vi "APC_9049_MODBUSTCP_HealingLoop.vi"() -> ()   [LabVIEW 2020]
doc: "This example demonstrates the procedure required to apply different NI-DAQmx Custom Scales to each virtual channel in a task. A DAQmx Task Property Node (Functions >> NI Measurements >> DAQmx - Data Acquisition >> DAQmx Advanced Task Options) is used to obtain the task's virtual channels. A DAQmx Channel Property Node (Functions >> NI Measurements >> DAQmx - Data Acquisition) is then used to set the custom scale for each virtual channel in the task.\n\nThe \"DAQmx Create Scale\" VI creates a custom scale for each channel in the channel list. *Note, make sure your Minimum and Maximum channel parameters are consistent with the range the scale will create."
uses:
  <vilib>/Modbus/master/Create Master Instance (TCP).vi
  <vilib>/Modbus/master/Modbus Master.lvclass
panel:
  in  "Slave address":string="172.22.11.1"
  out "register values":u16[](array[numeric])
  out "coil values":bool[](array[boolean])
  in  "Modbus STOP":bool
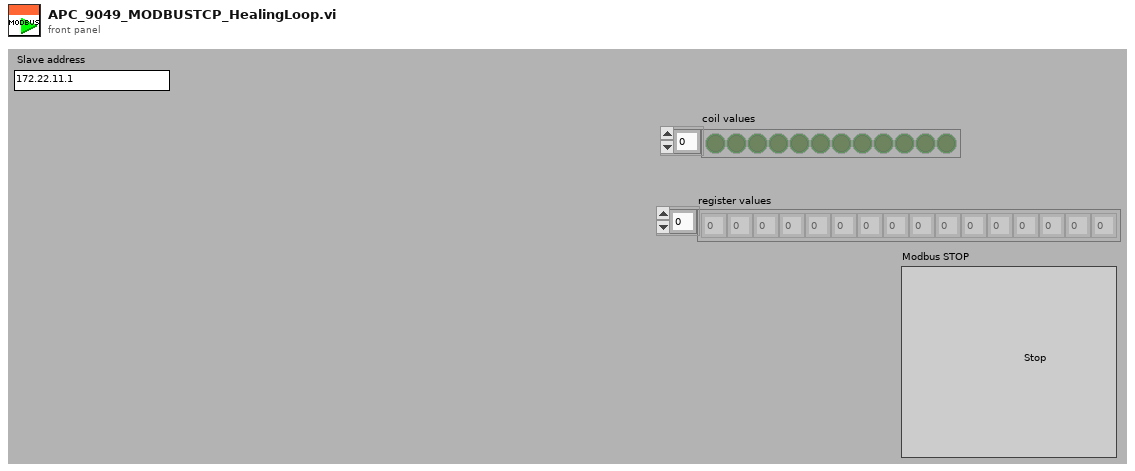
[diagram p1: front panel]
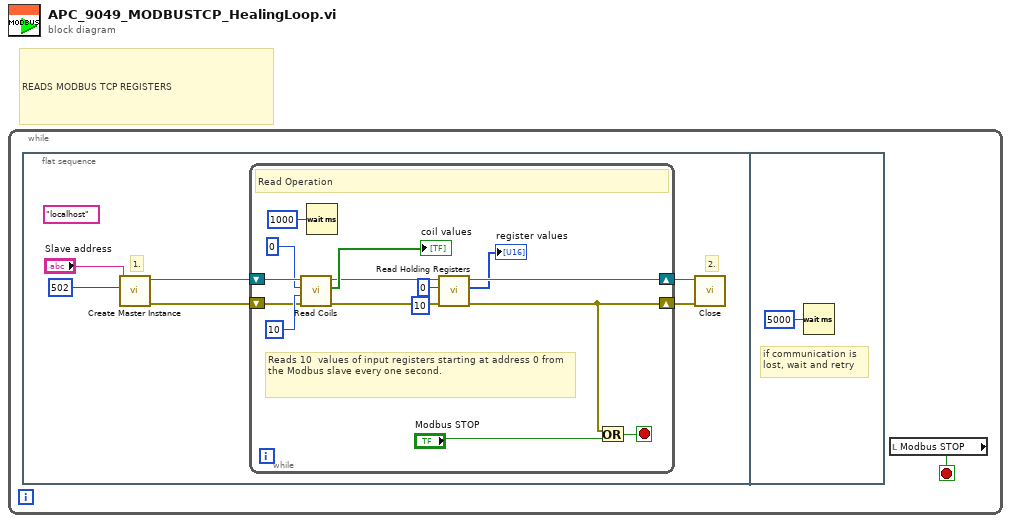
[diagram p0: block diagram]
diagram:
  # "READS MODBUS TCP REGISTERS"
  n1 = while {
    stop <- w1 stop-if-true
    n2 = flat-sequence {
      frame #0 {
        (unwired) "localhost" ("address")
        # "1."
        # "2."
        n3 = call-poly <vilib>:"Create Master Instance.vi"("port (502)"=u16 502, "address"="Slave address") -> ("error out"=w2:errorcluster, "TCP master instance"=w3:refnum<class "Modbus Master.lvclass">)  [unwired: 8 in]
        n4 = while {
          shift-right: [w11] -> w7
          shift-left: w2 -> [w19]
          shift-right: [w12] -> w6
          shift-left: w3 -> [w20]
          stop <- w16 stop-if-true
          # "Reads 10  values of input registers starting at address 0 from the Modbus slave every one second."
          # "Read Operation"
          n5 = call-dynamic "Read Coils.vi"("error in (no error)"=w19, "number of coils"=u16 10 ("number of inputs"), "starting address"=u16 0, "Modbus master in"=w20) -> ("error out"=w13:errorcluster, "coil values"=→"coil values":bool[], "Modbus master out"=w14:refnum<class "Modbus Master.lvclass">)  [unwired: 5 in]
          n6 = Wait (ms)(milliseconds to wait=u32 1000) -> ()  [unwired: 1 out]
          n7 = call-dynamic "Read Holding Registers.vi"("error in (no error)"=w13, "number of holding registers"=u16 10, "starting address"=u16 0, "Modbus master in"=w14) -> ("error out"=w11:errorcluster, "register values"=→"register values":u16[], "Modbus master out"=w12:refnum<class "Modbus Master.lvclass">)  [unwired: 5 in]
          n8 = Or(x=w11, y="Modbus STOP") -> (x .or. y?=w16:bool)
        }
        n9 = call-dynamic "Close.vi"("error in (no error)"=w7, "Modbus master in"=w6) -> ()  [unwired: 9 in, 1 out]
      }
      frame #1 {
        # "if communication is lost, wait and retry"
        n10 = Wait (ms)(milliseconds to wait=u32 5000) -> ()  [unwired: 1 out]
      }
    }
    n11 = local read "Modbus STOP"() -> (w1:bool)
  }
